vi "Save Load Shooter Settings.vi"(8 "error in":errorcluster, 10 "Shooter Settings (in)":T1, 11 "Save Load Info":T3) -> (0 "error out":errorcluster, 2 "Shooter Settings(out)":T1, 3 "Save Load Info (out)":T3)   [LabVIEW 2016]
uses:
  Load Save Info.ctl
  <vilib>/Utility/config.llb/Config Data RefNum.ctl
  Shooter Settings.ctl
  PID Settings.ctl
  <vilib>/Utility/config.llb/NI_LVConfig.lvlib
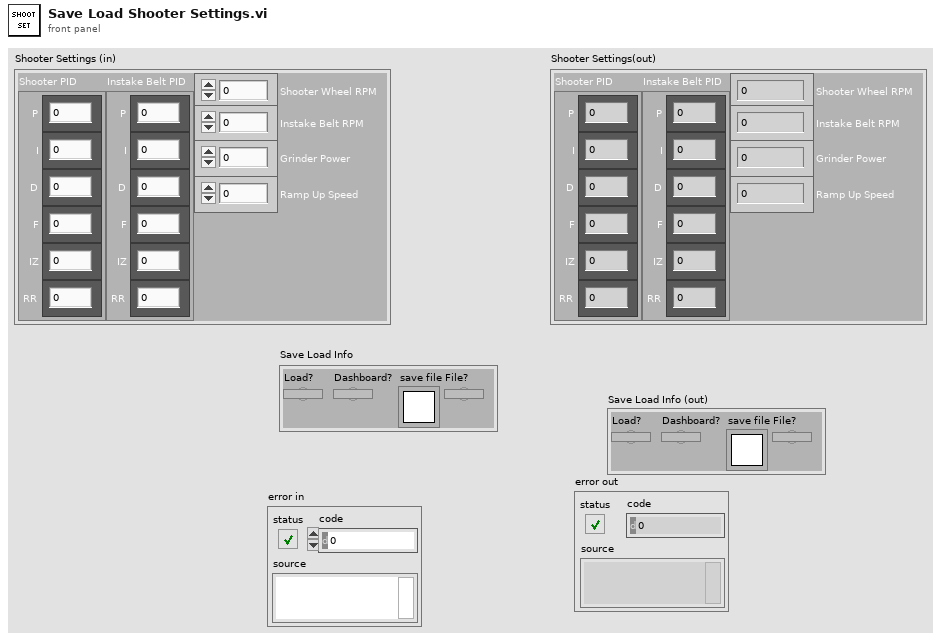
[diagram p1: front panel]
types:
  T1 = typedef "Shooter Settings.ctl" = cluster{"Shooter PID":T2, "Instake Belt PID":T2, "Shooter Wheel RPM":dbl, "Instake Belt RPM":dbl, "Grinder Power":dbl, "Ramp Up Speed":dbl}
  T2 = typedef "PID Settings.ctl" = cluster{"D":dbl, "F":dbl, "RR":dbl, "IZ":dbl, "P":dbl, "I":dbl}
  T3 = typedef "Load Save Info.ctl" = cluster{"Load?":bool, "Dashboard?":bool, "save file":T4, "File?":bool}
  T4 = typedef "NI_LVConfig.lvlib/Config Data RefNum.ctl" = refnum<k1>
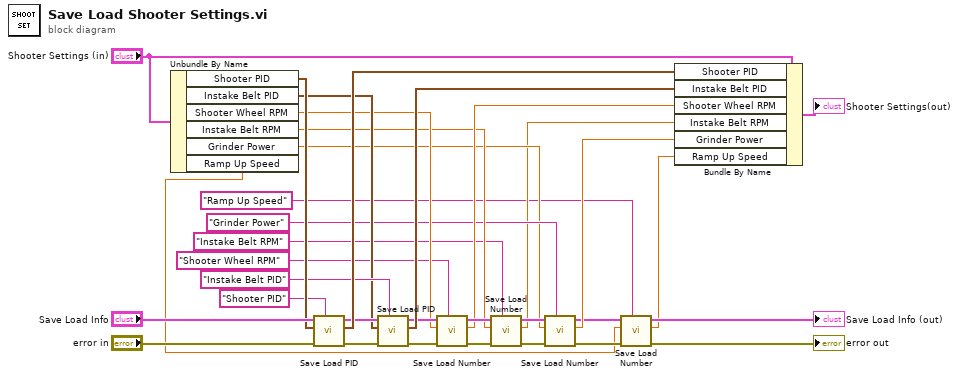
[diagram p0: block diagram]
diagram:
  n1 = Unbundle By Name("Shooter Settings (in)") -> ("Shooter PID"=w31:T2, "Instake Belt PID"=w24:T2, "Shooter Wheel RPM"=w16:dbl, "Instake Belt RPM"=w13:dbl, "Grinder Power"=w10:dbl, "Ramp Up Speed"=w2:dbl)
  n2 = call "Save Load PID.vi"("Name"="Shooter PID", "error in"="error in", "PID (in)"=w31, "Save Load Info (in)"="Save Load Info") -> ("error out"=w26:errorcluster, "PID (out)"=w30:T2, "Save Load Info (out)"=w27:T3)  [unwired: 5 in]
  n3 = call "Save Load PID.vi"("Name"="Instake Belt PID", "error in"=w26, "PID (in)"=w24, "Save Load Info (in)"=w27) -> ("error out"=w17:errorcluster, "PID (out)"=w23:T2, "Save Load Info (out)"=w18:T3)  [unwired: 5 in]
  n4 = call "Save Load Number.vi"("Name"="Shooter Wheel RPM", "error in"=w17, "Num (in)"=w16, "Save Load Info (in)"=w18) -> ("error out"=w22:errorcluster, "Num (out)"=w15:dbl, "Save Load Info (out)"=w21:T3)  [unwired: 5 in]
  n5 = call "Save Load Number.vi"("Name"="Instake Belt RPM", "error in"=w22, "Num (in)"=w13, "Save Load Info (in)"=w21) -> ("error out"=w20:errorcluster, "Num (out)"=w8:dbl, "Save Load Info (out)"=w19:T3)  [unwired: 5 in]
  n6 = call "Save Load Number.vi"("Name"="Grinder Power", "error in"=w20, "Num (in)"=w10, "Save Load Info (in)"=w19) -> ("error out"=w5:errorcluster, "Num (out)"=w9:dbl, "Save Load Info (out)"=w7:T3)  [unwired: 5 in]
  n7 = call "Save Load Number.vi"("Name"="Ramp Up Speed", "error in"=w5, "Num (in)"=w2, "Save Load Info (in)"=w7) -> ("error out"=→"error out":errorcluster, "Num (out)"=w1:dbl, "Save Load Info (out)"=→"Save Load Info (out)":T3)  [unwired: 5 in]
  n8 = Bundle By Name(cluster="Shooter Settings (in)", "Shooter PID"=w30, "Instake Belt PID"=w23, "Shooter Wheel RPM"=w15, "Instake Belt RPM"=w8, "Grinder Power"=w9, "Ramp Up Speed"=w1) -> (→"Shooter Settings(out)":T1)
